vi "HSSS mcc.vi"() -> ()   [LabVIEW 2021]
panel:
  out "concatenated string":string
  out "hex integer string":string
  out "length":i32
  in  "Array":sgl[](array[numeric])
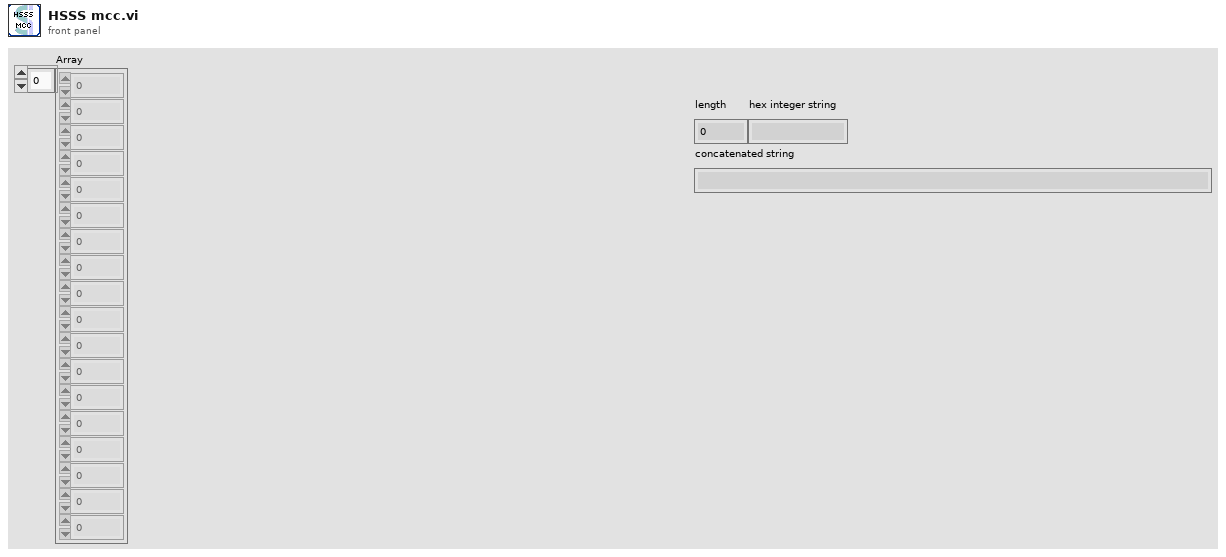
[diagram p1: front panel]
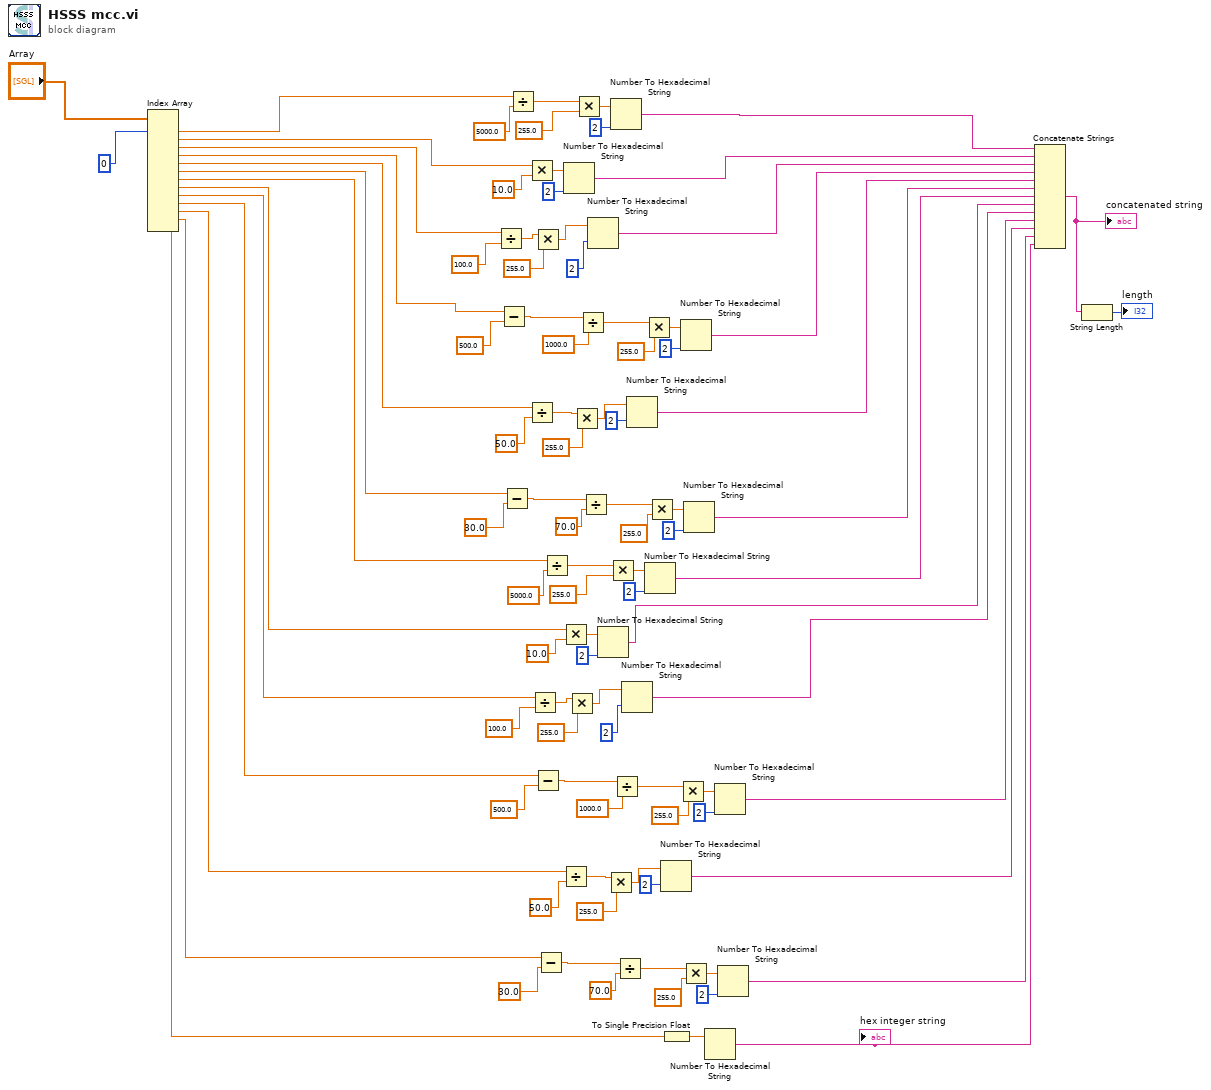
[diagram p0: block diagram]
diagram:
  n1 = Index Array(array="Array", index #1=0 ("index")) -> (element #1=w53:sgl, element #2=w51:sgl, element #3=w66:sgl, element #4=w73:sgl, element #5=w78:sgl, element #6=w85:sgl, element #7=w17:sgl, element #8=w16:sgl, element #9=w15:sgl, element #10=w14:sgl, element #11=w13:sgl, element #12=w12:sgl, element #13=w2:sgl)  [unwired: 12 in]
  n2 = Divide(x=w66, y=100.0) -> (x/y=w63:dbl)
  n3 = Subtract(x=w73, y=500.0) -> (x-y=w67:dbl)
  n4 = Subtract(x=w85, y=30.0) -> (x-y=w84:dbl)
  n5 = Divide(x=w53, y=sgl 5000.0) -> (x/y=w59:sgl)
  n6 = Multiply(x=w51, y=sgl 10.0) -> (x*y=w56:sgl)
  n7 = Divide(x=w78, y=50.0) -> (x/y=w75:dbl)
  n8 = Divide(x=w15, y=100.0) -> (x/y=w42:dbl)
  n9 = Multiply(x=w63, y=255.0) -> (x*y=w62:dbl)
  n10 = Subtract(x=w14, y=500.0) -> (x-y=w39:dbl)
  n11 = Subtract(x=w12, y=30.0) -> (x-y=w24:dbl)
  n12 = Divide(x=w17, y=5000.0) -> (x/y=w46:dbl)
  n13 = Multiply(x=w16, y=10.0) -> (x*y=w49:dbl)
  n14 = Divide(x=w13, y=50.0) -> (x/y=w32:dbl)
  n15 = Number To Hexadecimal String(1:i16 2 ("width (-)"), 2:w56) -> (0:w50:string)
  n16 = Multiply(x=w42, y=255.0) -> (x*y=w43:dbl)
  n17 = Multiply(x=w75, y=255.0) -> (x*y=w74:dbl)
  n18 = Multiply(x=w59, y=sgl 255.0) -> (x*y=w58:sgl)
  n19 = Divide(x=w67, y=1000.0) -> (x/y=w69:dbl)
  n20 = Divide(x=w84, y=70.0) -> (x/y=w80:dbl)
  n21 = Number To Hexadecimal String(1:i16 2 ("width (-)"), 2:w62) -> (0:w86:string)
  n22 = Number To Hexadecimal String(1:i16 2 ("width (-)"), 2:w49) -> (0:w10:string)
  n23 = Multiply(x=w32, y=255.0) -> (x*y=w33:dbl)
  n24 = Multiply(x=w46, y=255.0) -> (x*y=w47:dbl)
  n25 = Number To Hexadecimal String(1:i16 2 ("width (-)"), 2:w58) -> (0:w52:string)
  n26 = Divide(x=w39, y=1000.0) -> (x/y=w37:dbl)
  n27 = Divide(x=w24, y=70.0) -> (x/y=w28:dbl)
  n28 = Number To Hexadecimal String(1:i16 2 ("width (-)"), 2:w43) -> (0:w9:string)
  n29 = Number To Hexadecimal String(1:i16 2 ("width (-)"), 2:w74) -> (0:w88:string)
  n30 = Multiply(x=w69, y=255.0) -> (x*y=w68:dbl)
  n31 = Number To Hexadecimal String(1:i16 2 ("width (-)"), 2:w47) -> (0:w11:string)
  n32 = Multiply(x=w80, y=255.0) -> (x*y=w82:dbl)
  n33 = Number To Hexadecimal String(1:i16 2 ("width (-)"), 2:w33) -> (0:w7:string)
  n34 = To Single Precision Float(number=w2) -> (single precision float=w3:sgl)
  n35 = Multiply(x=w37, y=255.0) -> (x*y=w38:dbl)
  n36 = Number To Hexadecimal String(1:i16 2 ("width (-)"), 2:w68) -> (0:w87:string)
  n37 = Multiply(x=w28, y=255.0) -> (x*y=w26:dbl)
  n38 = Number To Hexadecimal String(1:i16 2 ("width (-)"), 2:w82) -> (0:w89:string)
  n39 = Number To Hexadecimal String(2:w3) -> (0:w4:string)  [unwired: 1 in]
  "hex integer string" <- w4
  n40 = Number To Hexadecimal String(1:i16 2 ("width (-)"), 2:w38) -> (0:w8:string)
  n41 = Number To Hexadecimal String(1:i16 2 ("width (-)"), 2:w26) -> (0:w6:string)
  n42 = Concatenate Strings(w52, w50, w86, w87, w88, w89, w11, w10, w9, w8, w7, w6, w4) -> (w1:string)
  "concatenated string" <- w1
  n43 = String Length(string=w1) -> (length=→"length":i32)
